vi "SAC-Plot Response.vi"(0 "Cal.Data in":T1, 11 "error in (no error)":errorcluster) -> (4 "Cal.Data out":T1, 6 "time":cluster{"offset":dbl, "dx":dbl, "Y":dbl[]}, 8 "crosscorr":cluster{"offset":dbl, "dx":dbl, "Y":dbl[]}, 13 "phase":cluster{"offset":dbl, "dx":dbl, "Y":dbl[]}, 14 "mag":cluster{"offset":dbl, "dx":dbl, "Y":dbl[]}, 15 "error out":errorcluster)   [LabVIEW 2020]
uses:
  Typedefs/SAC-Runtime Data.ctl
  <vilib>/Analysis/2dsp.llb/Complex FFT.vi
  <vilib>/Analysis/2dsp.llb/Inverse Real FFT.vi
  Utility VIs/Math VIs/FFT x(t) to dB,Degrees (1D).vi
  Utility VIs/Conversion VIs/Create Waveform Cluster (1D).vi
  <vilib>/Analysis/NI_AALPro.lvlib
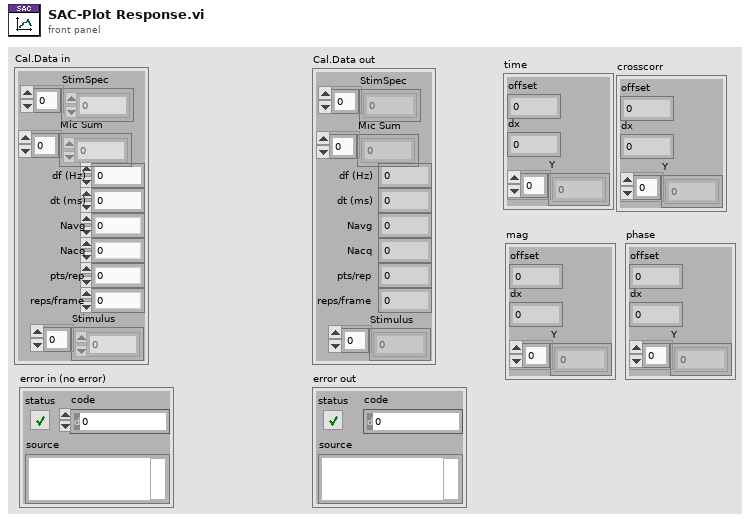
[diagram p1: front panel]
types:
  T1 = typedef "SAC-Runtime Data.ctl" = cluster{"StimSpec":cdb[], "Mic Sum":dbl[], "df (Hz)":dbl, "dt (ms)":dbl, "Navg":i32, "Nacq":i32, "pts/rep":i32, "reps/frame":i32, "Stimulus":dbl[]}
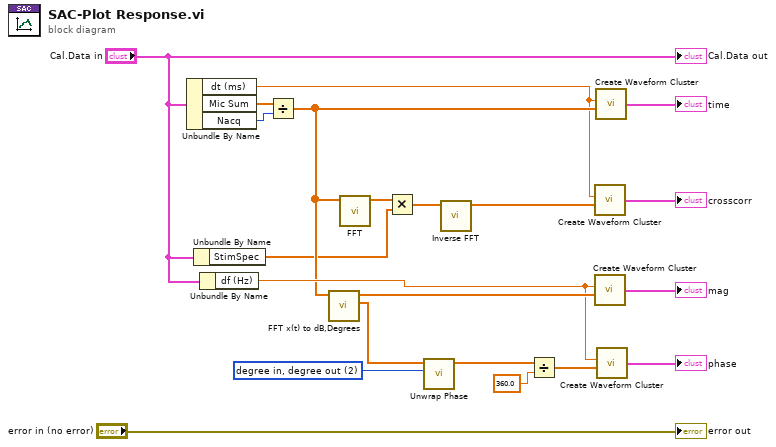
[diagram p0: block diagram]
diagram:
  w14 = 2 items=["radian in, radian out", "radian in, degree out", "degree in, degree out", "degree in, radian out"] ("phase unit")
  n1 = Unbundle By Name("Cal.Data in") -> ("dt (ms)"=w6:dbl, "Mic Sum"=w16:dbl[], "Nacq"=w15:i32)
  n2 = Unbundle By Name("Cal.Data in") -> ("StimSpec"=w5:cdb[])
  n3 = Unbundle By Name("Cal.Data in") -> ("df (Hz)"=w9:dbl)
  n4 = Divide(x=w16, y=w15) -> (x/y=w8:dbl[])
  n5 = call-poly "FFT x(t) to dB,Degrees.vi"("X"=w8) -> ("+Freq Phase of FFT (degrees)"=w3:dbl[], "+Freq. Mag of FFT (dB rms)"=w12:dbl[])  [unwired: 8 in, 1 out]
  n6 = call-poly <vilib>:"FFT.vi"("X"=w8) -> ("FFT {X}"=w2:cdb[])  [unwired: 9 in, 1 out]
  n7 = Multiply(x=w2, y=w5) -> (x*y=w1:cdb[])
  n8 = call <vilib>:"Unwrap Phase.vi"("phase unit"=w14, "Phase"=w3) -> ("Unwrapped Phase"=w11:dbl[])  [unwired: 8 in, 1 out]
  n9 = call-poly <vilib>:"Inverse FFT.vi"("FFT {X}"=w1) -> ("X"=w7:dbl[])  [unwired: 9 in, 1 out]
  n10 = Divide(x=w11, y=360.0) -> (x/y=w10:dbl[])
  n11 = call-poly "Create Waveform Cluster.vi"("dx"=w6, "Y"=w7) -> ("waveform cluster"=→"crosscorr":cluster{dbl, "dx":dbl, "Y":dbl[]})  [unwired: 3 in]
  n12 = call-poly "Create Waveform Cluster.vi"("dx"=w9, "Y"=w12) -> ("waveform cluster"=→"mag":cluster{dbl, "dx":dbl, "Y":dbl[]})  [unwired: 3 in]
  n13 = call-poly "Create Waveform Cluster.vi"("dx"=w6, "Y"=w8) -> ("waveform cluster"=→"time":cluster{dbl, "dx":dbl, "Y":dbl[]})  [unwired: 3 in]
  n14 = call-poly "Create Waveform Cluster.vi"("dx"=w9, "Y"=w10) -> ("waveform cluster"=→"phase":cluster{dbl, "dx":dbl, "Y":dbl[]})  [unwired: 3 in]
  "error out" <- "error in (no error)"
  "Cal.Data out" <- "Cal.Data in"
